vi "Flush Message Queue.vi"(8 "Error In":errorcluster) -> (0 "Error Out":errorcluster, 3 "Remaining Messages":T1[](array[typedef]))   [LabVIEW 2023, in "QSM - Library.lvlib"]
doc: "This VI flushes the message queue and returns the remaining messages for the Queued State Machine template."
uses:
  QSM - Library.lvlib
  Controls/Message Queue Element.ctl
  Controls/State Machine Message.ctl
  Controls/Message Queue Reference Functional Global Variable Operation.ctl
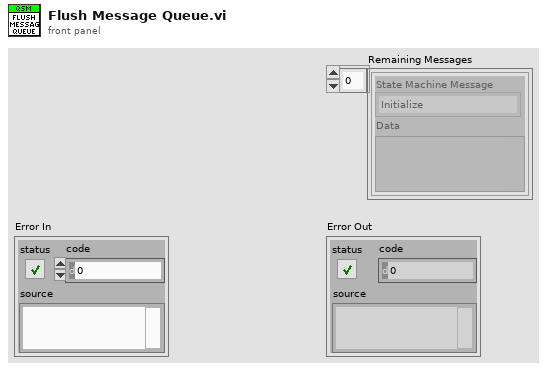
[diagram p1: front panel]
types:
  T1 = typedef "QSM - Library.lvlib/Message Queue Element.ctl" = cluster{"State Machine Message":T2, "Data":variant}
  T2 = typedef "QSM - Library.lvlib/State Machine Message.ctl" = enum16{"Initialize", "Handle Error", "Exit"}
  T3 = typedef "QSM - Library.lvlib/Message Queue Reference Functional Global Variable Operation.ctl" = enum16{"Set", "Get"}
  T4 = typedef "QSM - Library.lvlib/Message Queue Reference.ctl" = refnum<queue>
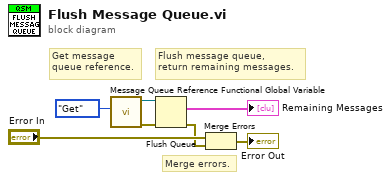
[diagram p0: block diagram]
diagram:
  # "Merge errors."
  # "Flush message queue,\nreturn remaining messages."
  # "Get message\nqueue reference."
  n1 = call "Message Queue Reference Functional Global Variable.vi"("Operation"=Message_Queue_Reference_Functional_Global_Variable_Operation."Get") -> ("Error Out"=w7:errorcluster, "Message Queue Reference Out"=w6:T4)  [unwired: 9 in]
  n2 = Flush Queue(queue=w6, error in (no error)=w7) -> (remaining elements=→"Remaining Messages":T1[], error out=w2:errorcluster)  [unwired: 1 out]
  n3 = Merge Errors("Error In", w2) -> (→"Error Out":errorcluster)
